vi "ODE-Generator.vi"(6 "error in (no error)":errorcluster, 9 "Cluster":T1) -> (0 "error out":errorcluster, 1 "Final ODE 2":string[](array[string]), 2 "Final ODE":string[](array[string]), 3 "SP-for-ODE":string[](array[string]))   [LabVIEW 2014]
panel:
  out "Math-w/-ch-VarID Output":string[](array[string])
  out "Output Laws":string[](array[string])
  out "Comp IDs":string[](array[string])
  out "OnlySubstanceUnits":string[](array[string])
  out "Intr_Kinetic_Law 2":string
  out "Math-w/-ch-VarID":string[](array[string])
  out "R-Stoich-for ODE":string[](array[string])
  out "P-Stoich-for ODE":string[](array[string])
  out "P-Stoich-separate":string[](array[string])
  out "R-Stoich-separate":string[](array[string])
  out "Bound Cond ODE SP":string[](array[string])
  out "Sp_Id_Arr":string[](array[string])
  out "Bound Cond":string[](array[string])
  out "P-Stoich":string[](array[string])
  out "Kinetic Laws":string[](array[string])
  out "Products":string[](array[string])
  out "R-Stoich":string[](array[string])
  out "Reactants":string[](array[string])
  out "Intr_Kinetic_Law":string
  out "R-Sp-for-ODE":string[](array[string])
  out "P-SP-for-ODE":string[](array[string])
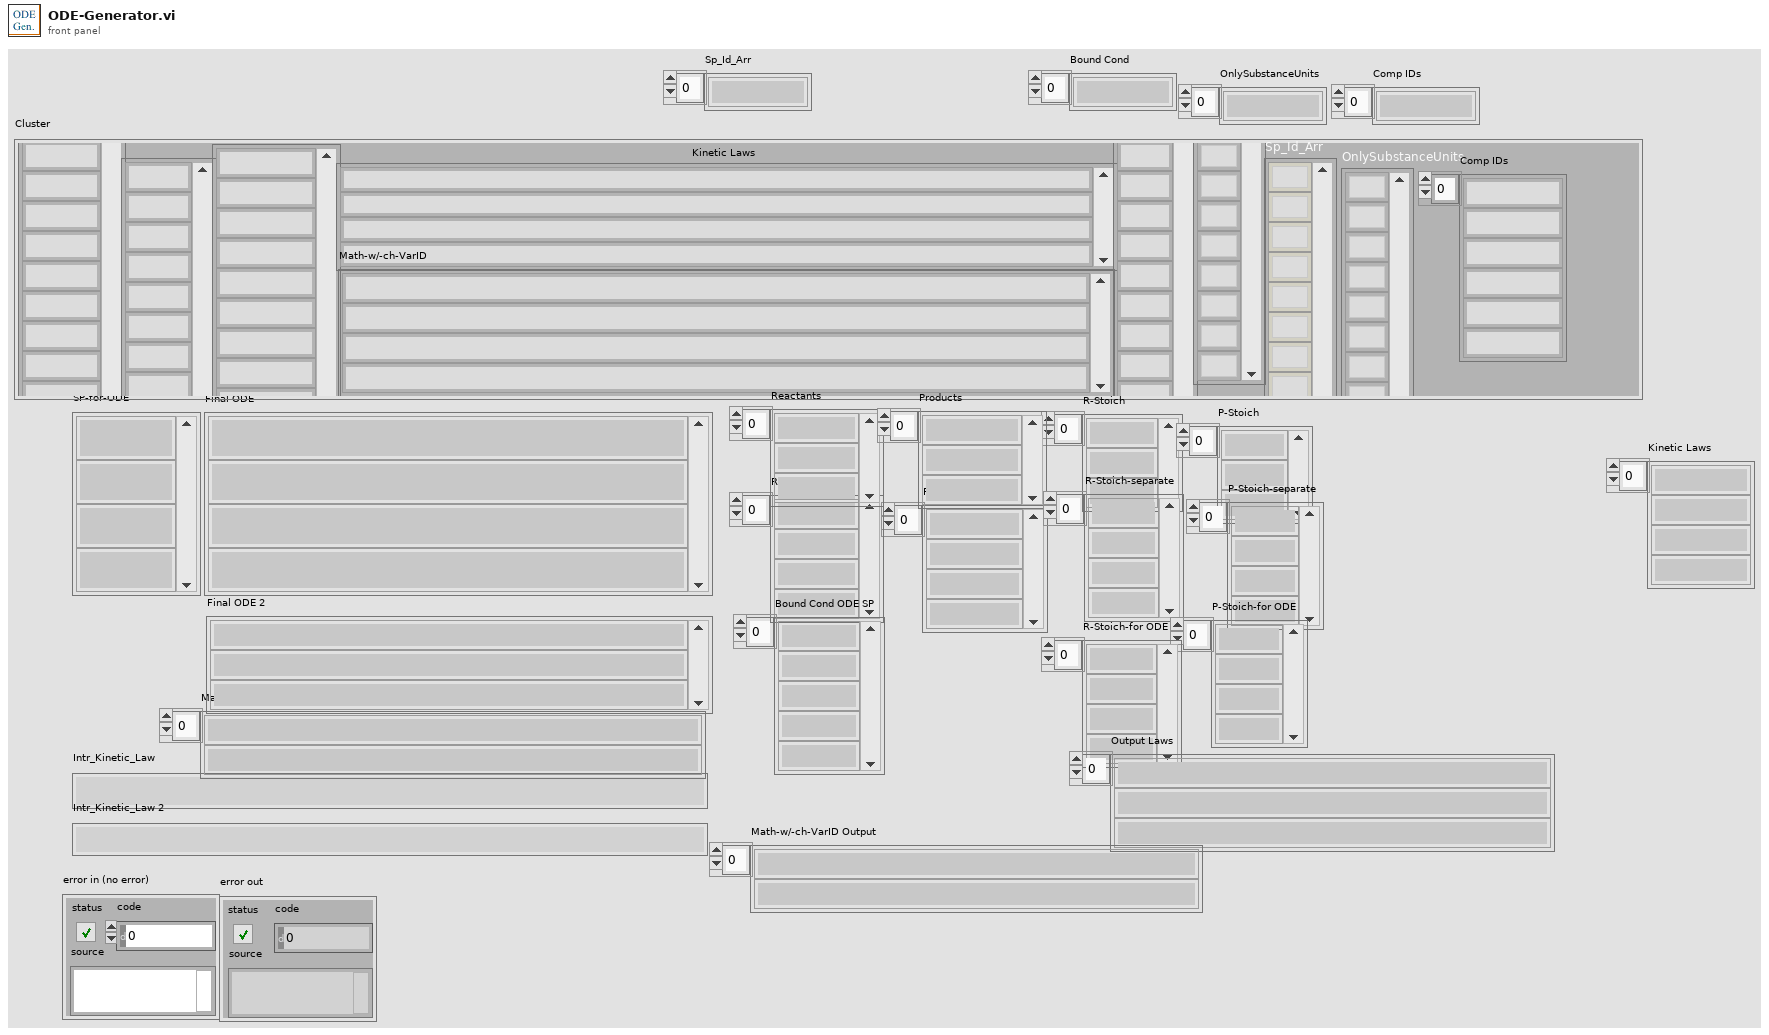
[diagram p1: front panel]
types:
  T1 = cluster{"Reactants":string[], "R-Stoich":string[], "Products":string[], "Kinetic Laws":string[], "P-Stoich":string[], "Bound Cond":string[], "Sp_Id_Arr":string[], "Math-w/-ch-VarID":string[], "OnlySubstanceUnits":string[], "Comp IDs":string[]}
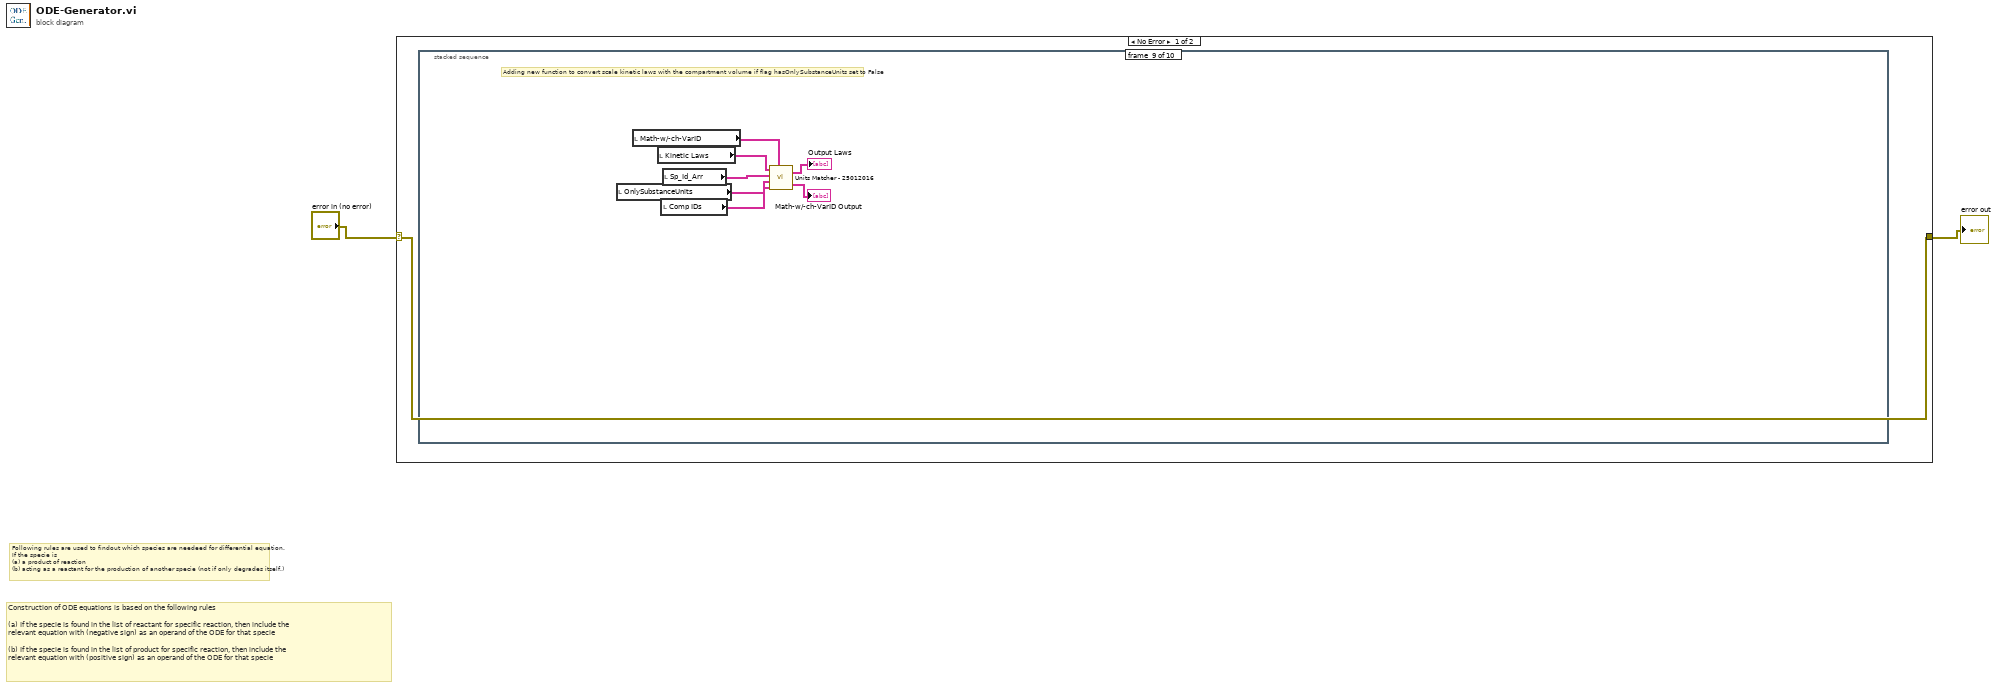
[diagram p0: block diagram]
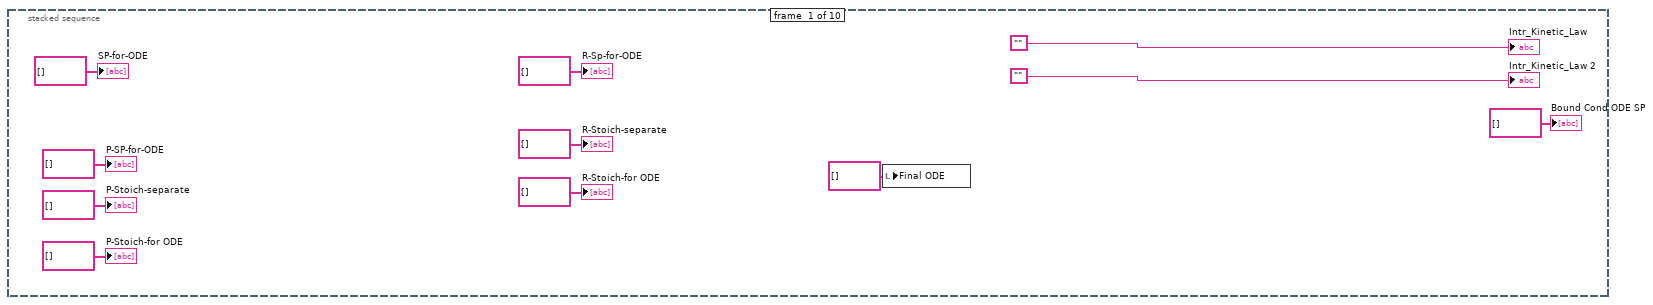
[diagram p2: hidden frame]
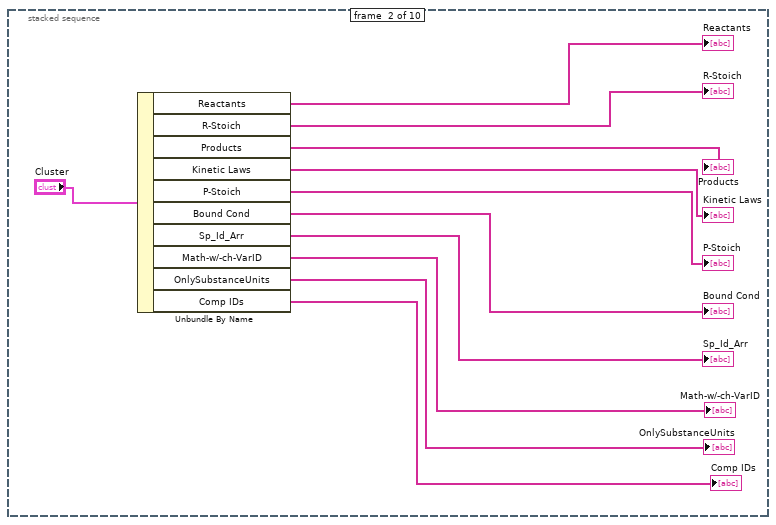
[diagram p3: hidden frame]
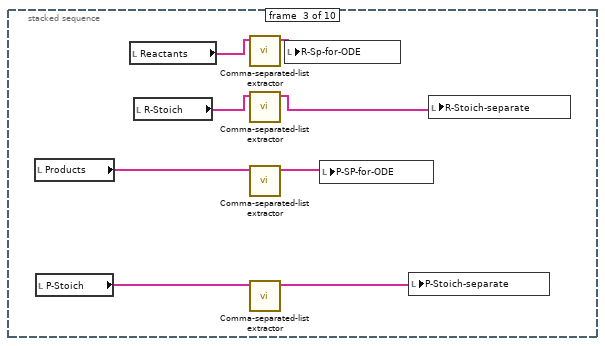
[diagram p4: hidden frame]
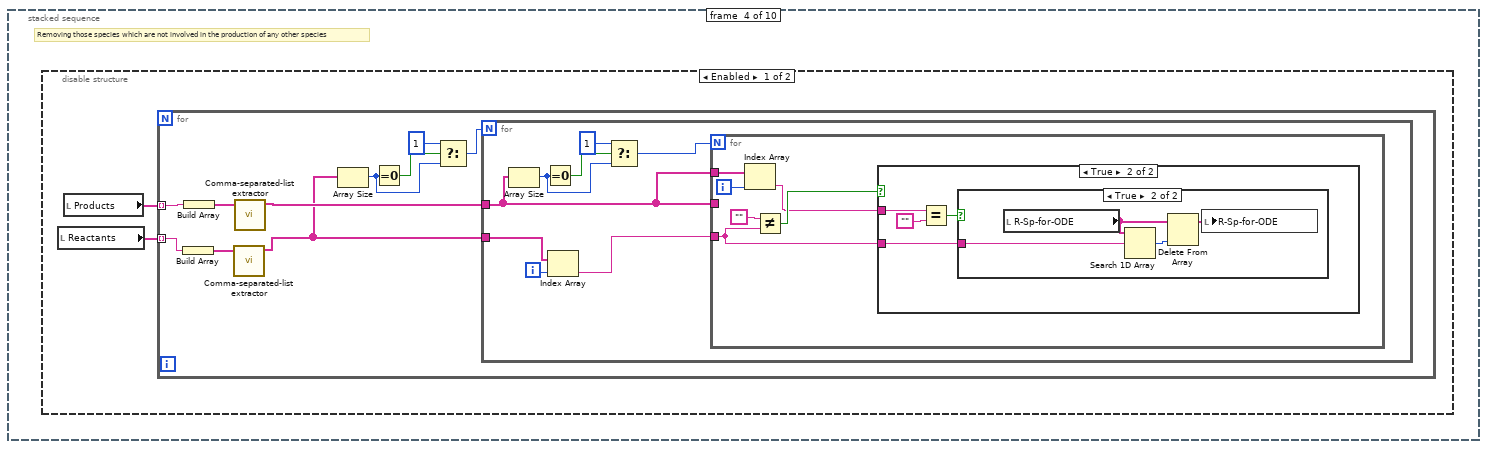
[diagram p5: hidden frame]
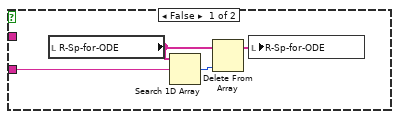
[diagram p6: hidden frame]
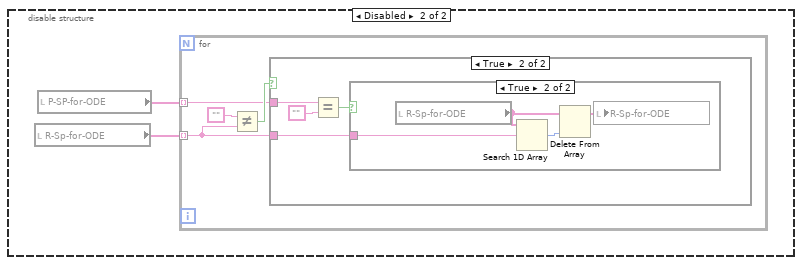
[diagram p8: hidden frame]
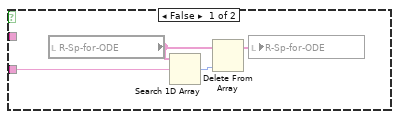
[diagram p9: hidden frame]
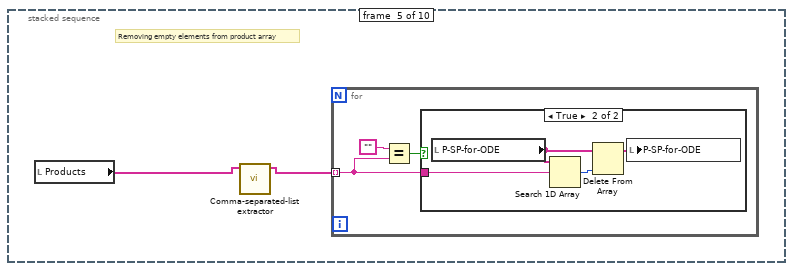
[diagram p11: hidden frame]
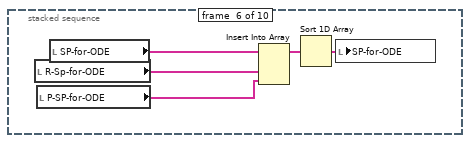
[diagram p13: hidden frame]
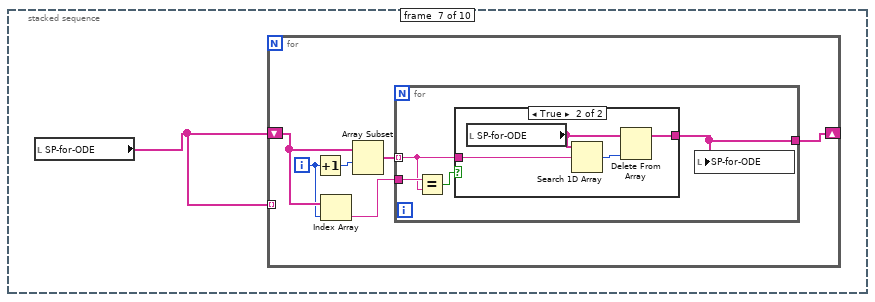
[diagram p14: hidden frame]
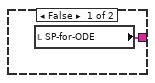
[diagram p15: hidden frame]
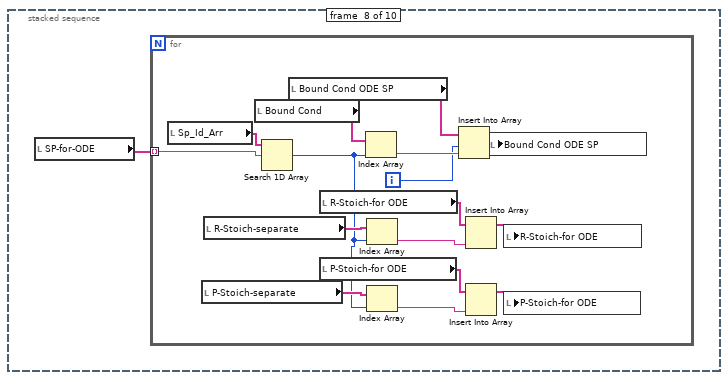
[diagram p16: hidden frame]
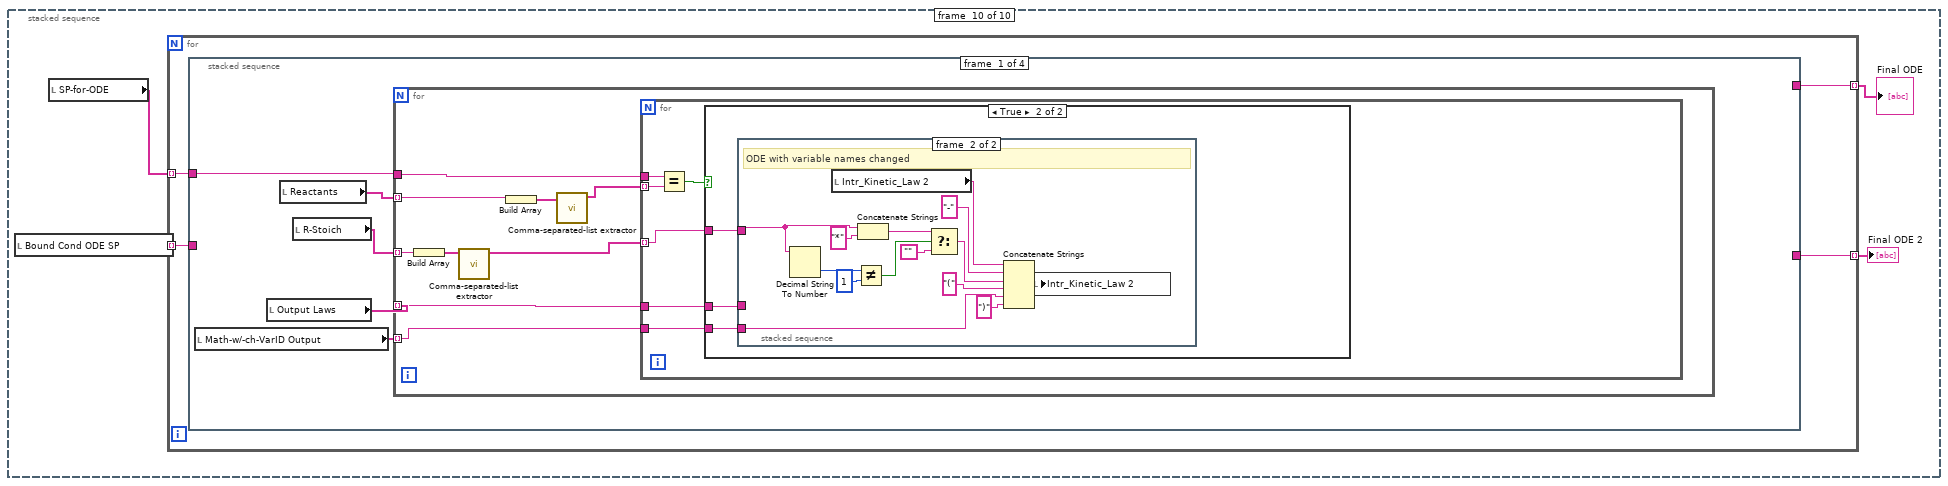
[diagram p17: hidden frame]
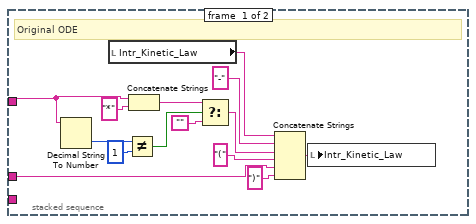
[diagram p19: hidden frame]
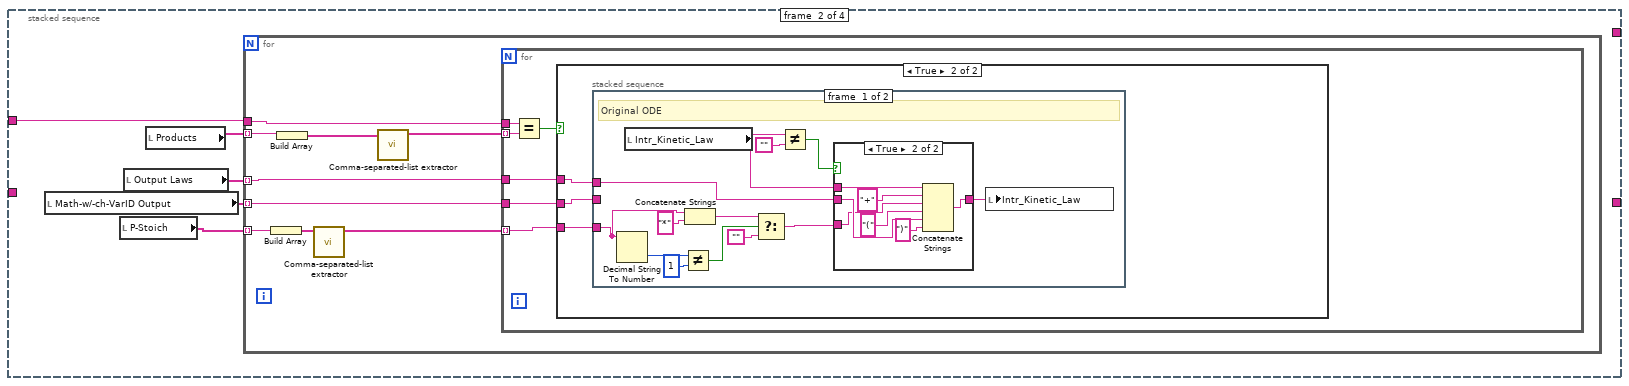
[diagram p20: hidden frame]
diagram:
  # "Construction of ODE equations is based on the following rules\n\n(a) If the specie is found in the list of reactant for specific reaction, then include the \nrelevant equation with (negative sign) as an operand of the ODE for that specie\n\n(b) If the specie is found in the list of product for specific reaction, then include the \nrelevant equation with (positive sign) as an operand of the ODE for that specie"
  # "Following rules are used to findout which species are needeed for differential equation.\nIf the specie is \n(a) a product of reaction\n(b) acting as a reactant for the production of another specie (not if only degrades itself.)"
  n1 = case shown="No Error" "error in (no error)" {
    selector: "error in (no error)" -> [w3 w286]
    tunnel: [w3 w286] -> w1
    frame No Error {
      n2 = stacked-sequence {
        frame #0 {
          n3 = local write "Final ODE"(string[] [] ("Final ODE")) -> ()
          "SP-for-ODE" <- string[] [] ("output array")
          "P-SP-for-ODE" <- string[] [] ("output array")
          "R-Sp-for-ODE" <- string[] [] ("output array")
          "Intr_Kinetic_Law" <- ""
          "Bound Cond ODE SP" <- string[] [] ("Bound Cond ODE SP")
          "R-Stoich-separate" <- string[] [] ("output array")
          "P-Stoich-separate" <- string[] [] ("output array")
          "P-Stoich-for ODE" <- string[] [] ("output array")
          "R-Stoich-for ODE" <- string[] [] ("output array")
          "Intr_Kinetic_Law 2" <- ""
        }
        frame #1 {
          n4 = Unbundle By Name("Cluster") -> ("Reactants"=→"Reactants":string[], "R-Stoich"=→"R-Stoich":string[], "Products"=→"Products":string[], "Kinetic Laws"=→"Kinetic Laws":string[], "P-Stoich"=→"P-Stoich":string[], "Bound Cond"=→"Bound Cond":string[], "Sp_Id_Arr"=→"Sp_Id_Arr":string[], "Math-w/-ch-VarID"=→"Math-w/-ch-VarID":string[], "OnlySubstanceUnits"=→"OnlySubstanceUnits":string[], "Comp IDs"=→"Comp IDs":string[])
        }
        frame #2 {
          n5 = local read "Products"() -> (w30:string[])
          n6 = local read "P-Stoich"() -> (w28:string[])
          n7 = local read "Reactants"() -> (w33:string[])
          n8 = local read "R-Stoich"() -> (w31:string[])
          n9 = call "Comma-separated-list extractor.vi"("In_list"=w33) -> ("List_Out"=w32:string[])  [unwired: 6 in, 1 out]
          n10 = call "Comma-separated-list extractor.vi"("In_list"=w31) -> ("List_Out"=w27:string[])  [unwired: 6 in, 1 out]
          n11 = call "Comma-separated-list extractor.vi"("In_list"=w30) -> ("List_Out"=w29:string[])  [unwired: 6 in, 1 out]
          n12 = call "Comma-separated-list extractor.vi"("In_list"=w28) -> ("List_Out"=w26:string[])  [unwired: 6 in, 1 out]
          n13 = local write "R-Sp-for-ODE"(w32) -> ()
          n14 = local write "P-SP-for-ODE"(w29) -> ()
          n15 = local write "P-Stoich-separate"(w26) -> ()
          n16 = local write "R-Stoich-separate"(w27) -> ()
        }
        frame #3 {
          # "Removing those species which are not involved in the production of any other species"
          n17 = disable-structure shown="Enabled" {
            frame Enabled {
              n18 = local read "Reactants"() -> (w35:string[])
              n19 = local read "Products"() -> (w34:string[])
              n20 = for {
                tunnel: w35 -> [w41] mode=indexing
                tunnel: w34 -> [w44] mode=indexing
                n21 = Build Array(w41) -> (w42:string[])
                n22 = Build Array(w44) -> (w45:string[])
                n23 = call "Comma-separated-list extractor.vi"("In_list"=w42) -> ("List_Out"=w37:string[])  [unwired: 6 in, 1 out]
                n24 = call "Comma-separated-list extractor.vi"("In_list"=w45) -> ("List_Out"=w43:string[])  [unwired: 6 in, 1 out]
                n25 = Array Size(array=w37) -> (size(s)=w39:i32)
                n26 = Equal To 0?(x=w39) -> (x = 0?=w38:bool)
                n27 = Select(t=1, s=w38, f=w39) -> (s? t:f=w36:i32)
                n28 = for {
                  N: w36 -> [_]
                  tunnel: w37 -> [w47]
                  tunnel: w43 -> [w49]
                  i -> [w48]
                  n29 = Array Size(array=w49) -> (size(s)=w52:i32)
                  n30 = Equal To 0?(x=w52) -> (x = 0?=w53:bool)
                  n31 = Index Array(array=w47, index=w48) -> (element=w46:string)
                  n32 = Select(t=1, s=w53, f=w52) -> (s? t:f=w50:i32)
                  n33 = for {
                    N: w50 -> [_]
                    tunnel: w46 -> [w57]
                    tunnel: w49 -> [_]
                    tunnel: w49 -> [w56]
                    i -> [w55]
                    n34 = Index Array(array=w56, index=w55) -> (element=w54:string)
                    n35 = Not Equal?(x="", y=w57) -> (x != y?=w59:bool)
                    n36 = case shown="True" w59 {
                      tunnel: w54 -> [_ w66]
                      tunnel: w57 -> [w60 w64]
                      frame False {
                        n37 = local read "R-Sp-for-ODE"() -> (w63:string[])
                        n38 = Search 1D Array(1D array=w63, element=w60) -> (index of element=w62:i32)  [unwired: 1 in]
                        n39 = Delete From Array(array=w63, index=w62) -> (array with subset deleted=w61:string[])  [unwired: 1 in, 1 out]
                        n40 = local write "R-Sp-for-ODE"(w61) -> ()
                      }
                      frame True {
                        n41 = Equal?(x=w66, y="") -> (x = y?=w65:bool)
                        n42 = case shown="True" w65 {
                          tunnel: w64 -> [_ w71]
                          frame False {
                          }
                          frame True {
                            n43 = local read "R-Sp-for-ODE"() -> (w70:string[])
                            n44 = Search 1D Array(1D array=w70, element=w71) -> (index of element=w69:i32)  [unwired: 1 in]
                            n45 = Delete From Array(array=w70, index=w69) -> (array with subset deleted=w68:string[])  [unwired: 1 in, 1 out]
                            n46 = local write "R-Sp-for-ODE"(w68) -> ()
                          }
                        }
                      }
                    }
                  }
                }
              }
            }
            frame Disabled {
              n47 = local read "R-Sp-for-ODE"() -> (w73:string[])
              n48 = local read "P-SP-for-ODE"() -> (w72:string[])
              n49 = for {
                tunnel: w73 -> [w74] mode=indexing
                tunnel: w72 -> [w76] mode=indexing
                n50 = Not Equal?(x="", y=w74) -> (x != y?=w77:bool)
                n51 = case shown="True" w77 {
                  tunnel: w76 -> [_ w84]
                  tunnel: w74 -> [w78 w82]
                  frame False {
                    n52 = local read "R-Sp-for-ODE"() -> (w81:string[])
                    n53 = Search 1D Array(1D array=w81, element=w78) -> (index of element=w80:i32)  [unwired: 1 in]
                    n54 = Delete From Array(array=w81, index=w80) -> (array with subset deleted=w79:string[])  [unwired: 1 in, 1 out]
                    n55 = local write "R-Sp-for-ODE"(w79) -> ()
                  }
                  frame True {
                    n56 = Equal?(x=w84, y="") -> (x = y?=w83:bool)
                    n57 = case shown="True" w83 {
                      tunnel: w82 -> [_ w89]
                      frame False {
                      }
                      frame True {
                        n58 = local read "R-Sp-for-ODE"() -> (w88:string[])
                        n59 = Search 1D Array(1D array=w88, element=w89) -> (index of element=w87:i32)  [unwired: 1 in]
                        n60 = Delete From Array(array=w88, index=w87) -> (array with subset deleted=w86:string[])  [unwired: 1 in, 1 out]
                        n61 = local write "R-Sp-for-ODE"(w86) -> ()
                      }
                    }
                  }
                }
              }
            }
          }
        }
        frame #4 {
          # "Removing empty elements from product array"
          n62 = local read "Products"() -> (w91:string[])
          n63 = call "Comma-separated-list extractor.vi"("In_list"=w91) -> ("List_Out"=w90:string[])  [unwired: 6 in, 1 out]
          n64 = for {
            tunnel: w90 -> [w92] mode=indexing
            n65 = Equal?(x="", y=w92) -> (x = y?=w93:bool)
            n66 = case shown="True" w93 {
              tunnel: w92 -> [_ w98]
              frame False {
              }
              frame True {
                n67 = local read "P-SP-for-ODE"() -> (w97:string[])
                n68 = Search 1D Array(1D array=w97, element=w98) -> (index of element=w96:i32)  [unwired: 1 in]
                n69 = Delete From Array(array=w97, index=w96) -> (array with subset deleted=w95:string[])  [unwired: 1 in, 1 out]
                n70 = local write "P-SP-for-ODE"(w95) -> ()
              }
            }
          }
        }
        frame #5 {
          n71 = local read "R-Sp-for-ODE"() -> (w102:string[])
          n72 = local read "P-SP-for-ODE"() -> (w101:string[])
          n73 = local read "SP-for-ODE"() -> (w103:string[])
          n74 = Insert Into Array(array=w103, new element #1=w102, new element #2=w101) -> (w100:string[])  [unwired: 1 in]
          n75 = Sort 1D Array(array=w100) -> (sorted array=w99:string[])
          n76 = local write "SP-for-ODE"(w99) -> ()
        }
        frame #6 {
          n77 = local read "SP-for-ODE"() -> (w104:string[])
          n78 = for {
            shift-right: [w108] -> _
            shift-left: w104 -> [w107]
            tunnel: w104 -> [_] mode=indexing
            i -> [w106]
            n79 = Increment(x=w106) -> (x+1=w110:i32)
            n80 = Index Array(array=w107, index=w106) -> (element=w105:string)
            n81 = Array Subset(array=w107, index=w110) -> (w109:string[])  [unwired: 1 in]
            n82 = for {
              tunnel: w109 -> [w112] mode=indexing
              tunnel: w105 -> [w114]
              tunnel: [w111] -> w108
              n83 = Equal?(x=w114, y=w112) -> (x = y?=w113:bool)
              n84 = case shown="True" w113 {
                tunnel: [w115 w119] -> w111
                tunnel: w112 -> [_ w116]
                frame False {
                  n85 = local read "SP-for-ODE"() -> (w115:string[])
                }
                frame True {
                  n86 = local read "SP-for-ODE"() -> (w118:string[])
                  n87 = Search 1D Array(1D array=w118, element=w116) -> (index of element=w117:i32)  [unwired: 1 in]
                  n88 = Delete From Array(array=w118, index=w117) -> (array with subset deleted=w119:string[])  [unwired: 1 in, 1 out]
                }
              }
              n89 = local write "SP-for-ODE"(w111) -> ()
            }
          }
        }
        frame #7 {
          n90 = local read "SP-for-ODE"() -> (w120:string[])
          n91 = for {
            tunnel: w120 -> [w135] mode=indexing
            i -> [w130]
            n92 = local read "Sp_Id_Arr"() -> (w136:string[])
            n93 = local read "P-Stoich-separate"() -> (w122:string[])
            n94 = local read "R-Stoich-separate"() -> (w129:string[])
            n95 = local read "Bound Cond"() -> (w134:string[])
            n96 = Search 1D Array(1D array=w136, element=w135) -> (index of element=w121:i32)  [unwired: 1 in]
            n97 = local read "Bound Cond ODE SP"() -> (w131:string[])
            n98 = local read "R-Stoich-for ODE"() -> (w127:string[])
            n99 = local read "P-Stoich-for ODE"() -> (w124:string[])
            n100 = Index Array(array=w134, index=w121) -> (element=w133:string)
            n101 = Index Array(array=w129, index=w121) -> (element=w128:string)
            n102 = Index Array(array=w122, index=w121) -> (element=w123:string)
            n103 = Insert Into Array(array=w131, index=w130, new element=w133) -> (w132:string[])
            n104 = Insert Into Array(array=w127, new element=w128) -> (w126:string[])  [unwired: 1 in]
            n105 = Insert Into Array(array=w124, new element=w123) -> (w125:string[])  [unwired: 1 in]
            n106 = local write "Bound Cond ODE SP"(w132) -> ()
            n107 = local write "R-Stoich-for ODE"(w126) -> ()
            n108 = local write "P-Stoich-for ODE"(w125) -> ()
          }
        }
        frame #8 {
          # "Adding new function to convert scale kinetic laws with the compartment volume if flag hasOnlySubstanceUnits set to False"
          n109 = local read "OnlySubstanceUnits"() -> (w141:string[])
          n110 = local read "Math-w/-ch-VarID"() -> (w138:string[])
          n111 = local read "Kinetic Laws"() -> (w143:string[])
          n112 = local read "Comp IDs"() -> (w140:string[])
          n113 = local read "Sp_Id_Arr"() -> (w142:string[])
          n114 = call "Units Matcher - 25012016.vi"("Math-w/-ch-VarID"=w138, "Comp IDs"=w140, "OnlySubstanceUnits"=w141, "Sp_Id_Arr"=w142, "Kinetic Laws"=w143) -> ("Math-w/-ch-VarID Output"=→"Math-w/-ch-VarID Output":string[], "Output Laws"=→"Output Laws":string[])  [unwired: 1 in]
        }
        frame #9 {
          n115 = local read "Bound Cond ODE SP"() -> (w145:string[])
          n116 = local read "SP-for-ODE"() -> (w147:string[])
          n117 = for {
            tunnel: w147 -> [w151] mode=indexing
            tunnel: [w150] -> w146 mode=indexing
            tunnel: w145 -> [w149] mode=indexing
            tunnel: [w148] -> w144 mode=indexing
            n118 = stacked-sequence {
              tunnel: w151 -> [w156 w206 _ _]
              tunnel: [_ _ w279 _] -> w150
              tunnel: w149 -> [_ _ w280 _]
              tunnel: [_ _ w276 _] -> w148
              frame #0 {
                n119 = local read "Math-w/-ch-VarID Output"() -> (w152:string[])
                n120 = local read "Output Laws"() -> (w155:string[])
                n121 = local read "Reactants"() -> (w154:string[])
                n122 = local read "R-Stoich"() -> (w153:string[])
                n123 = for {
                  tunnel: w156 -> [w165]
                  tunnel: w155 -> [w164] mode=indexing
                  tunnel: w154 -> [w163] mode=indexing
                  tunnel: w153 -> [w160] mode=indexing
                  tunnel: w152 -> [w157] mode=indexing
                  n124 = Build Array(w160) -> (w159:string[])
                  n125 = call "Comma-separated-list extractor.vi"("In_list"=w159) -> ("List_Out"=w158:string[])  [unwired: 6 in, 1 out]
                  n126 = Build Array(w163) -> (w162:string[])
                  n127 = call "Comma-separated-list extractor.vi"("In_list"=w162) -> ("List_Out"=w161:string[])  [unwired: 6 in, 1 out]
                  n128 = for {
                    tunnel: w165 -> [w171]
                    tunnel: w161 -> [w170] mode=indexing
                    tunnel: w164 -> [w168]
                    tunnel: w158 -> [w167] mode=indexing
                    tunnel: w157 -> [w166]
                    n129 = Equal?(x=w171, y=w170) -> (x = y?=w169:bool)
                    n130 = case shown="True" w169 {
                      tunnel: w167 -> [_ w174]
                      tunnel: w168 -> [_ w173]
                      tunnel: w166 -> [_ w172]
                      frame False {
                      }
                      frame True {
                        n131 = stacked-sequence {
                          tunnel: w174 -> [w180 w194]
                          tunnel: w173 -> [w175 _]
                          tunnel: w172 -> [_ w189]
                          frame #0 {
                            # "Original ODE"
                            n132 = Decimal String To Number(string=w180) -> (number=w183:i32)  [unwired: 2 in, 1 out]
                            n133 = local read "Intr_Kinetic_Law"() -> (w184:string)
                            n134 = Not Equal?(x=w183, y=1) -> (x != y?=w181:bool)
                            n135 = Concatenate Strings(w180, "*" ("string")) -> (w178:string)
                            n136 = Select(t=w178, s=w181, f="") -> (s? t:f=w177:string)
                            n137 = Concatenate Strings(w184, "-" ("string"), w177, "(" ("string"), w175, ")" ("string")) -> (w185:string)
                            n138 = local write "Intr_Kinetic_Law"(w185) -> ()
                          }
                          frame #1 {
                            # "ODE with variable names changed"
                            n139 = Decimal String To Number(string=w194) -> (number=w197:i32)  [unwired: 2 in, 1 out]
                            n140 = local read "Intr_Kinetic_Law 2"() -> (w198:string)
                            n141 = Not Equal?(x=w197, y=1) -> (x != y?=w195:bool)
                            n142 = Concatenate Strings(w194, "*" ("string")) -> (w192:string)
                            n143 = Select(t=w192, s=w195, f="") -> (s? t:f=w191:string)
                            n144 = Concatenate Strings(w198, "-" ("string"), w191, "(" ("string"), w189, ")" ("string")) -> (w199:string)
                            n145 = local write "Intr_Kinetic_Law 2"(w199) -> ()
                          }
                        }
                      }
                    }
                  }
                }
              }
              frame #1 {
                n146 = local read "Math-w/-ch-VarID Output"() -> (w203:string[])
                n147 = local read "P-Stoich"() -> (w205:string[])
                n148 = local read "Output Laws"() -> (w204:string[])
                n149 = local read "Products"() -> (w207:string[])
                n150 = for {
                  tunnel: w207 -> [w213] mode=indexing
                  tunnel: w206 -> [w216]
                  tunnel: w205 -> [w210] mode=indexing
                  tunnel: w204 -> [w215] mode=indexing
                  tunnel: w203 -> [w208] mode=indexing
                  n151 = Build Array(w210) -> (w211:string[])
                  n152 = Build Array(w213) -> (w212:string[])
                  n153 = call "Comma-separated-list extractor.vi"("In_list"=w211) -> ("List_Out"=w209:string[])  [unwired: 6 in, 1 out]
                  n154 = call "Comma-separated-list extractor.vi"("In_list"=w212) -> ("List_Out"=w214:string[])  [unwired: 6 in, 1 out]
                  n155 = for {
                    tunnel: w216 -> [w222]
                    tunnel: w214 -> [w221] mode=indexing
                    tunnel: w209 -> [w219] mode=indexing
                    tunnel: w215 -> [w218]
                    tunnel: w208 -> [w217]
                    n156 = Equal?(x=w222, y=w221) -> (x = y?=w220:bool)
                    n157 = case shown="True" w220 {
                      tunnel: w219 -> [_ w225]
                      tunnel: w218 -> [_ w224]
                      tunnel: w217 -> [_ w223]
                      frame False {
                      }
                      frame True {
                        n158 = stacked-sequence {
                          tunnel: w225 -> [w227 w252]
                          tunnel: w224 -> [w226 _]
                          tunnel: w223 -> [_ w251]
                          frame #0 {
                            # "Original ODE"
                            n159 = Decimal String To Number(string=w227) -> (number=w234:i32)  [unwired: 2 in, 1 out]
                            n160 = local read "Intr_Kinetic_Law"() -> (w236:string)
                            n161 = Not Equal?(x=w234, y=1) -> (x != y?=w232:bool)
                            n162 = Concatenate Strings(w227, "*" ("string")) -> (w230:string)
                            n163 = Select(t=w230, s=w232, f="") -> (s? t:f=w228:string)
                            n164 = Not Equal?(x=w236, y="") -> (x != y?=w235:bool)
                            n165 = case shown="True" w235 {
                              tunnel: w226 -> [w241 w247]
                              tunnel: [w240 w246] -> w238
                              tunnel: w236 -> [_ w245]
                              tunnel: w228 -> [w242 w244]
                              frame False {
                                n166 = Concatenate Strings(w242, "(" ("string"), w241, ")" ("string")) -> (w240:string)
                              }
                              frame True {
                                n167 = Concatenate Strings(w245, "+" ("string"), w244, "(" ("string"), w247, ")" ("string")) -> (w246:string)
                              }
                            }
                            n168 = local write "Intr_Kinetic_Law"(w238) -> ()
                          }
                          frame #1 {
                            # "ODE with variable names changed"
                            n169 = local read "Intr_Kinetic_Law 2"() -> (w261:string)
                            n170 = Decimal String To Number(string=w252) -> (number=w259:i32)  [unwired: 2 in, 1 out]
                            n171 = Not Equal?(x=w259, y=1) -> (x != y?=w257:bool)
                            n172 = Concatenate Strings(w252, "*" ("string")) -> (w255:string)
                            n173 = Select(t=w255, s=w257, f="") -> (s? t:f=w253:string)
                            n174 = Not Equal?(x=w261, y="") -> (x != y?=w260:bool)
                            n175 = case shown="True" w260 {
                              tunnel: w251 -> [w266 w272]
                              tunnel: [w265 w271] -> w263
                              tunnel: w261 -> [_ w270]
                              tunnel: w253 -> [w267 w269]
                              frame False {
                                n176 = Concatenate Strings(w267, "(" ("string"), w266, ")" ("string")) -> (w265:string)
                              }
                              frame True {
                                n177 = Concatenate Strings(w270, "+" ("string"), w269, "(" ("string"), w272, ")" ("string")) -> (w271:string)
                              }
                            }
                            n178 = local write "Intr_Kinetic_Law 2"(w263) -> ()
                          }
                        }
                      }
                    }
                  }
                }
              }
              frame #2 {
                n179 = Equal?(x=w280, y="false") -> (x = y?=w277:bool)
                n180 = case shown="True" w277 {
                  tunnel: [w281 w283] -> w279
                  tunnel: [w281 w282] -> w276
                  frame False {
                    w281 = ""
                  }
                  frame True {
                    n181 = local read "Intr_Kinetic_Law 2"() -> (w282:string)
                    n182 = local read "Intr_Kinetic_Law"() -> (w283:string)
                  }
                }
              }
              frame #3 {
                n183 = local write "Intr_Kinetic_Law 2"("") -> ()
                n184 = local write "Intr_Kinetic_Law"("") -> ()
              }
            }
          }
          "Final ODE" <- w146
          "Final ODE 2" <- w144
        }
      }
    }
    frame Error {
    }
  }
  "error out" <- w1
